vi "Marker X Axes Values.vi"(8 "error in (no error)":errorcluster, 11 "VISA resource name":refnum<visa-resource-name>) -> (0 "error out":errorcluster, 1 "x Marker Value":dbl format="%^.3e", 2 "o Marker Value":dbl format="%^.3e", 3 "VISA resource name out":refnum<visa-resource-name>, 4 "o - x Diff Marker Value":dbl format="%.3f")   [LabVIEW 2010, in "Agilent 4194.lvlib"]
doc: "This function outputs the markers and cursors data valid for X axis."
uses:
  <instrlib>/Agilent 4194/Agilent 4194.lvlib
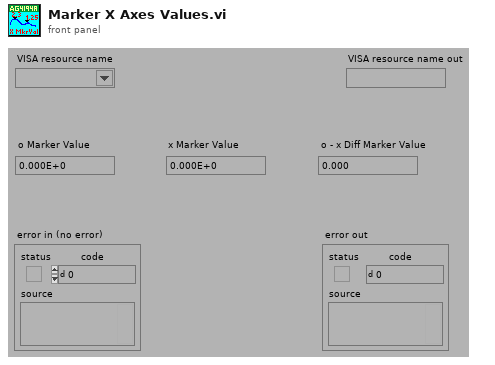
[diagram p1: front panel]
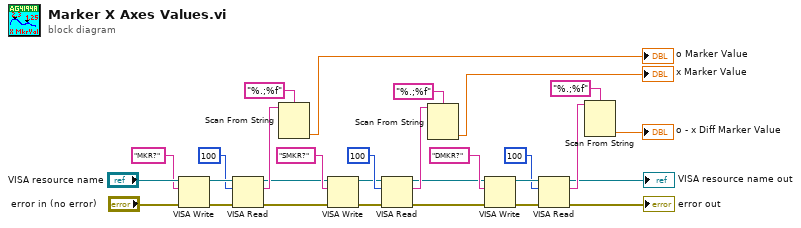
[diagram p0: block diagram]
diagram:
  n1 = VISA Write(VISA resource name="VISA resource name", write buffer="MKR?" ("write buffer (\"\")"), error in (no error)="error in (no error)") -> (VISA resource name out=w26:refnum<visa-resource-name>, error out=w27:errorcluster)  [unwired: 1 out]
  n2 = VISA Read(VISA resource name=w26, byte count=u32 100 ("byte count (0)"), error in (no error)=w27) -> (VISA resource name out=w10:refnum<visa-resource-name>, read buffer=w23:string, error out=w9:errorcluster)  [unwired: 1 out]
  n3 = Scan From String(format string="%.;%f", input string=w23) -> (output 1=→"o Marker Value":dbl)  [unwired: 3 in, 3 out]
  n4 = VISA Write(VISA resource name=w10, write buffer="SMKR?" ("write buffer (\"\")"), error in (no error)=w9) -> (VISA resource name out=w18:refnum<visa-resource-name>, error out=w17:errorcluster)  [unwired: 1 out]
  n5 = VISA Read(VISA resource name=w18, byte count=u32 100 ("byte count (0)"), error in (no error)=w17) -> (VISA resource name out=w8:refnum<visa-resource-name>, read buffer=w20:string, error out=w7:errorcluster)  [unwired: 1 out]
  n6 = Scan From String(format string="%.;%f", input string=w20) -> (output 1=→"x Marker Value":dbl)  [unwired: 3 in, 3 out]
  n7 = VISA Write(VISA resource name=w8, write buffer="DMKR?" ("write buffer (\"\")"), error in (no error)=w7) -> (VISA resource name out=w15:refnum<visa-resource-name>, error out=w16:errorcluster)  [unwired: 1 out]
  n8 = VISA Read(VISA resource name=w15, byte count=u32 100 ("byte count (0)"), error in (no error)=w16) -> (VISA resource name out=→"VISA resource name out":refnum<visa-resource-name>, read buffer=w13:string, error out=→"error out":errorcluster)  [unwired: 1 out]
  n9 = Scan From String(format string="%.;%f", input string=w13) -> (output 1=→"o - x Diff Marker Value":dbl)  [unwired: 3 in, 3 out]
